vi "Graph properties after stop.vi"(11 "Array":refnum<vi>[](array[refnum])) -> ()   [LabVIEW 2013]
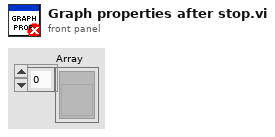
[diagram p1: front panel]
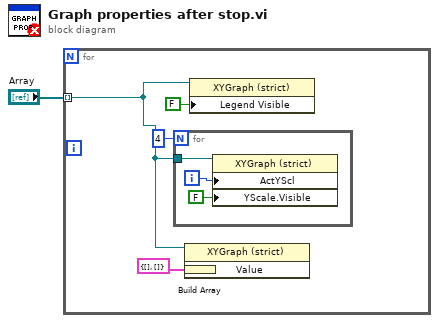
[diagram p0: block diagram]
diagram:
  n1 = for {
    tunnel: "Array" -> [w3] mode=indexing
    n2 = for {
      N: 4 -> [_]
      tunnel: w3 -> [w9]
      i -> [w8]
      n3 = property class="XYGraph (strict)"(reference=w9, "ActYScl"=w8, "YScale.Visible"=FALSE ("Y Scale.Visible")) -> ()  [unwired: 1 in, 2 out]
    }
    n4 = Build Array(cluster{timestamp[], dbl[]} {[], []} ("Graph i")) -> (w5:cluster{timestamp[], dbl[]}[])
    n5 = property on="Property Node" class="XYGraph (strict)"(reference=w3, "Value"=w5) -> ()  [unwired: 1 in, 2 out]
    n6 = property class="XYGraph (strict)"(reference=w3, "Legend Visible"=FALSE ("Legend:Visible")) -> ()  [unwired: 1 in, 2 out]
  }
